vi "Publish I32 Array.vi"(8 "error in (no error)":errorcluster, 10 "I32 Array":i32[](array[numeric]), 11 "MVC Subscription in":refnum<class "MVC Subscription.lvclass">) -> (0 "error out":errorcluster, 3 "MVC Subscription out":refnum<class "MVC Subscription.lvclass">)   [LabVIEW 2014, in "MVC Subscription.lvlib" / "MVC Subscription.lvclass"]
uses:
  MVC Subscription.lvclass
  MVC Subscription.lvclass/MVC Subscription.ctl
  Messages/Message (I32 Array)/_Message (I32 Array).lvclass
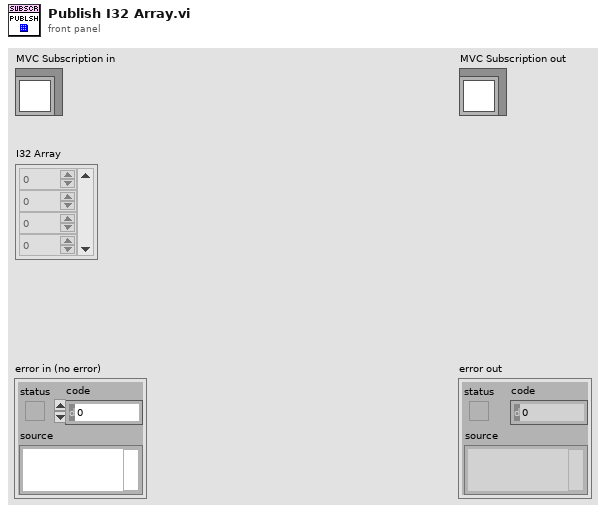
[diagram p1: front panel]
types:
  T1 = typedef "MVC Subscription.lvlib/MVC Subscription.lvclass/Cluster - Individual Subscription.ctl" = cluster{"Enqueuer":refnum<class "Message Enqueuer.lvclass">, "Message":refnum<class "Message.lvclass">}
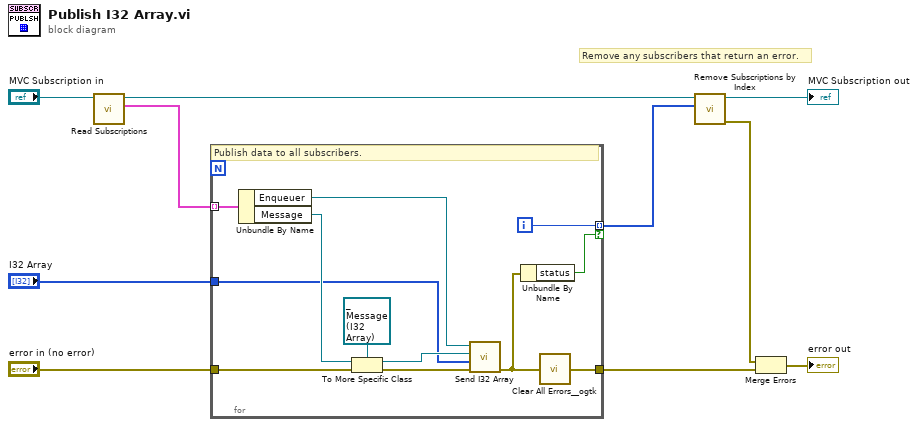
[diagram p0: block diagram]
diagram:
  # "Remove any subscribers that return an error."
  n1 = call "Read Subscriptions.vi"("MVC Subscription in"="MVC Subscription in") -> ("Subscriptions"=w6:T1[], "MVC Subscription out"=w8:refnum<class "MVC Subscription.lvclass">)  [unwired: 9 in]
  n2 = for {
    tunnel: "I32 Array" -> [w11]
    tunnel: w6 -> [w21] mode=indexing
    tunnel: "error in (no error)" -> [w22]
    tunnel: [w14] -> w2
    tunnel: [w13] -> w7 mode=indexing if=w12
    i -> [w13]
    # "Publish data to all subscribers."
    n3 = Unbundle By Name(w21) -> ("Enqueuer"=w20:refnum<class "Message Enqueuer.lvclass">, "Message"=w18:refnum<class "Message.lvclass">)
    n4 = To More Specific Class(target class=refnum<class "_Message (I32 Array).lvclass"> refnum ("_Message (I32).lvclass"), reference=w18, error in=w22) -> (specific class reference=w16:refnum<class "_Message (I32 Array).lvclass">, error out=w19:errorcluster)
    n5 = call-dynamic "Send I32 Array.vi"("error in"=w19, "I32 Array"=w11, "_Message (I32 Array) in"=w16, "Enqueuer"=w20) -> ("error out"=w15:errorcluster)  [unwired: 6 in, 1 out]
    n6 = Unbundle By Name(w15) -> ("status"=w12:bool)
    n7 = call <userlib>:"Clear All Errors__ogtk.vi"("Error In"=w15) -> ("Error Out"=w14:errorcluster)  [unwired: 3 in]
  }
  n8 = call "Remove Subscriptions by Index.vi"("Index of Elements to Remove"=w7, "MVC Subscription in"=w8) -> ("error out"=w3:errorcluster, "MVC Subscription out"=→"MVC Subscription out":refnum<class "MVC Subscription.lvclass">)  [unwired: 8 in]
  n9 = Merge Errors(w3, w2) -> (→"error out":errorcluster)
